vi "Disabled.vi"(7 "Robot Mode":T2, 10 "Match Info":T1={"Autonomous Elapsed Seconds"=0.0, "TeleOp Elapsed Seconds"=0.0, "Disabled Elapsed Seconds"=0.0, "Visited Autonomous"=FALSE, "Visited TeleOp"=FALSE, "Visited Disabled"=FALSE, "Autonomous Settings"={"Autonomous Style"=enum."Independent", "VI Refnum"=refnum}}, 11 "Call Context":T3) -> ()   [LabVIEW 2013]
doc: "This VI is called each time a disabled packet is received from the DS. It is often used to prepare for the next robot mode, to calibrate sensors, etc."
uses:
  <vilib>/Rock Robotics/WPI/DriverStation/WPI_DriverStationDerivedRobotMode.ctl
  <vilib>/Rock Robotics/WPI/DriverStation/WPI_DriverStationRobotMode2.ctl
  <vilib>/Rock Robotics/WPI/DriverStation/WPI_DriverStationMatch Info.ctl
  Systems/Catapult/Catapult.lvclass
  Systems/GrabberArms/GrabberArms.lvclass
  Systems/DriveMotors/DriveMotors.lvclass
  Robot Global Data.vi
panel:
  out "error out":errorcluster
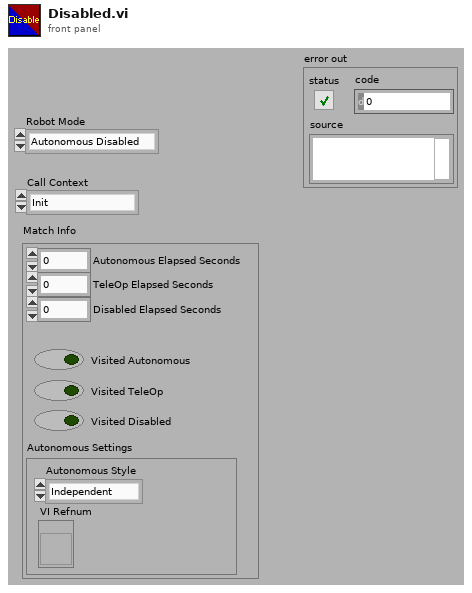
[diagram p1: front panel]
types:
  T1 = typedef "WPI_DriverStationMatch Info.ctl" = cluster{"Autonomous Elapsed Seconds":dbl, "TeleOp Elapsed Seconds":dbl, "Disabled Elapsed Seconds":dbl, "Visited Autonomous":bool, "Visited TeleOp":bool, "Visited Disabled":bool, "Autonomous Settings":cluster{"Autonomous Style":enum16{"Iterative", "Independent"}, "VI Refnum":refnum<vi>}}
  T2 = typedef "WPI_DriverStationRobotMode2.ctl" = enum16{"Autonomous Disabled", "Autonomous Enabled", "Teleop Disabled", "Teleop Enabled", "Timeout", "Finish", "Test Disabled", "Test Enabled"}
  T3 = typedef "WPI_DriverStationDerivedRobotMode.ctl" = enum16{"Init", "Execute", "Stop"}
  T4 = typedef "WPI_DriverStationAllianceInfo.ctl" = enum16{"Red", "Blue", "Invalid"}
  T5 = typedef "WPI_DigitalInputDevRef.ctl" = cluster{"DevStatus":errorcluster, "DIO Channel":T6, "Digital Module":T7}
  T6 = typedef "FPGA_DIOChannel.ctl" = enum8{"DIO 1", "DIO 2", "DIO 3", "DIO 4", "DIO 5", "DIO 6", "DIO 7", "DIO 8", "DIO 9", "DIO 10", "DIO 11", "DIO 12", "DIO 13", "DIO 14", "Invalid"}
  T7 = typedef "FPGA_TypedefDigitalModule.ctl" = enum16{"Digital Module 1", "Digital Module 2"}
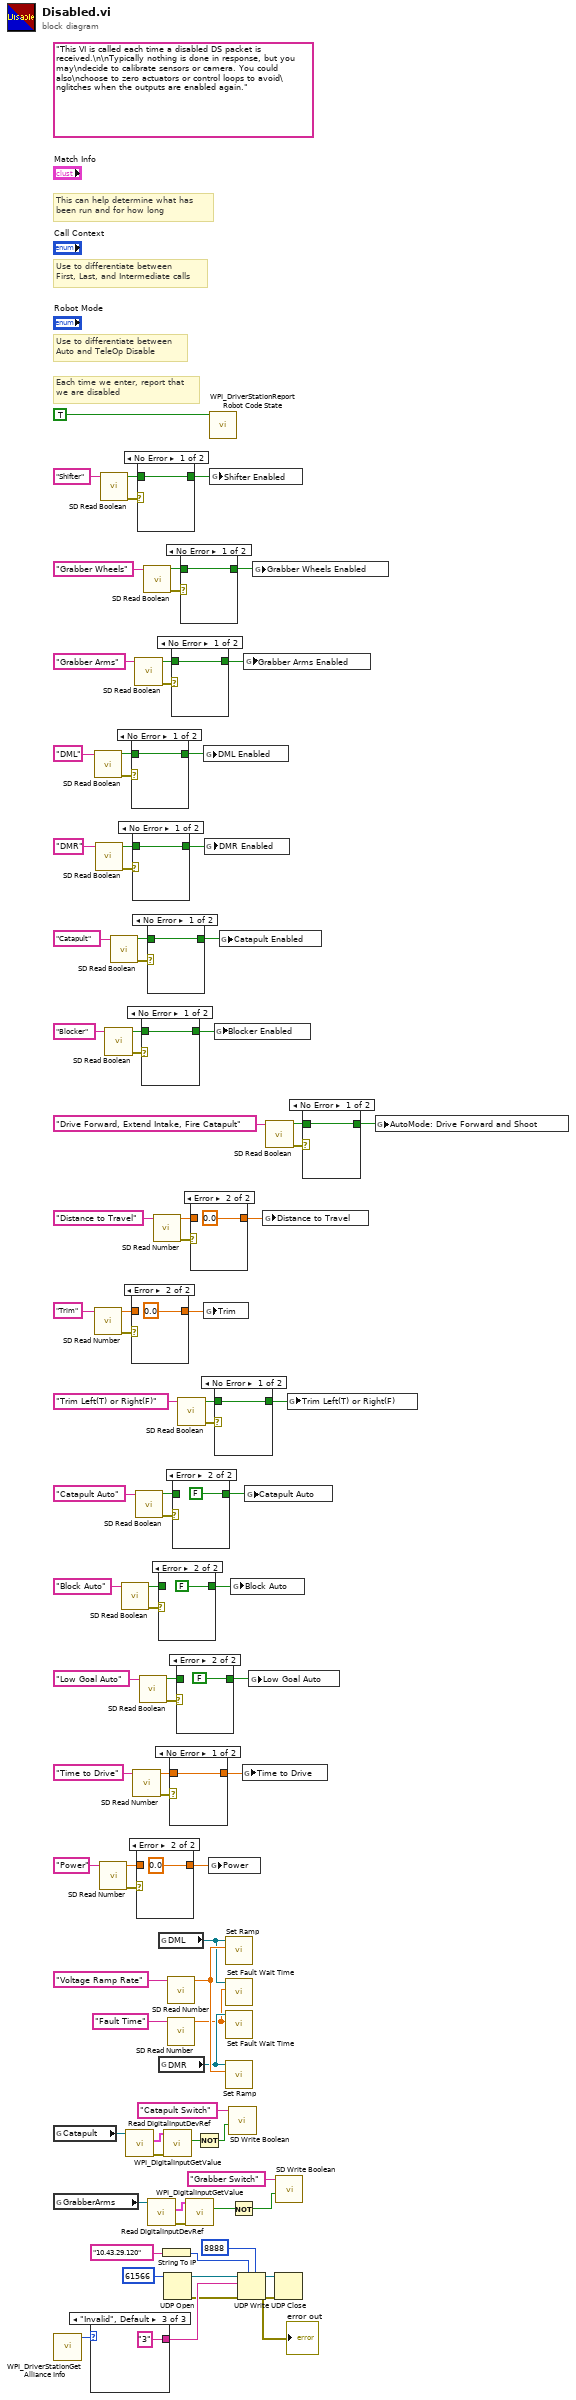
[diagram p0: block diagram]
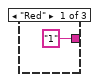
[diagram p2: hidden frame]
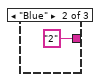
[diagram p3: hidden frame]
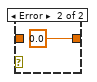
[diagram p8: hidden frame]
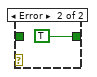
[diagram p9: hidden frame]
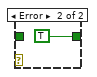
[diagram p12: hidden frame]
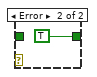
[diagram p13: hidden frame]
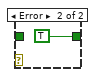
[diagram p14: hidden frame]
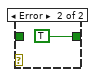
[diagram p15: hidden frame]
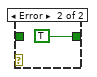
[diagram p16: hidden frame]
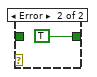
[diagram p17: hidden frame]
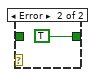
[diagram p18: hidden frame]
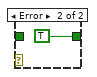
[diagram p19: hidden frame]
diagram:
  (unwired) "This VI is called each time a disabled DS packet is received.\n\nTypically nothing is done in response, but you may\ndecide to calibrate sensors or camera. You could also\nchoose to zero actuators or control loops to avoid\nglitches when the outputs are enabled again."
  # "Each time we enter, report that\nwe are disabled"
  # "Use to differentiate between\nFirst, Last, and Intermediate calls"
  # "This can help determine what has\nbeen run and for how long"
  # "Use to differentiate between\nAuto and TeleOp Disable"
  n1 = global read "Robot Global Data.vi" "Catapult"() -> (w39:refnum<class "Catapult.lvclass">)
  n2 = global read "Robot Global Data.vi" "GrabberArms"() -> (w5:refnum<class "GrabberArms.lvclass">)
  n3 = call <vilib>:"WPI_DriverStationGet Alliance Info.vi"() -> ("Alliance"=w11:T4)  [unwired: 10 in, 1 out]
  n4 = case shown="\"Invalid\", Default" w11 {
    tunnel: ["1" ("data in") "2" ("data in") "3" ("data in")] -> w10
    frame "Red" {
    }
    frame "Blue" {
    }
    frame "Invalid", Default {
    }
  }
  n5 = call <vilib>:"SD Read Boolean.vi"("Name"="DML") -> ("error out"=w83:errorcluster, "Boolean"=w74:bool)  [unwired: 8 in, 1 out]
  n6 = call <vilib>:"SD Read Number.vi"("Name"="Trim") -> ("error out"=w55:errorcluster, "Numeric"=w54:dbl)  [unwired: 8 in, 1 out]
  n7 = call <vilib>:"SD Read Boolean.vi"("Name"="DMR") -> ("error out"=w82:errorcluster, "Boolean"=w72:bool)  [unwired: 8 in, 1 out]
  n8 = call <vilib>:"SD Read Number.vi"("Name"="Power") -> ("error out"=w43:errorcluster, "Numeric"=w42:dbl)  [unwired: 8 in, 1 out]
  n9 = call <vilib>:"SD Read Boolean.vi"("Name"="Shifter") -> ("error out"=w86:errorcluster, "Boolean"=w80:bool)  [unwired: 8 in, 1 out]
  n10 = call <vilib>:"SD Read Boolean.vi"("Name"="Blocker") -> ("error out"=w66:errorcluster, "Boolean"=w67:bool)  [unwired: 8 in, 1 out]
  n11 = call <vilib>:"SD Read Boolean.vi"("Name"="Catapult") -> ("error out"=w81:errorcluster, "Boolean"=w70:bool)  [unwired: 8 in, 1 out]
  n12 = call <vilib>:"SD Read Boolean.vi"("Name"="Block Auto") -> ("error out"=w28:errorcluster, "Boolean"=w27:bool)  [unwired: 8 in, 1 out]
  n13 = call-dynamic "Read DigitalInputDevRef.vi"("Catapult in"=w39) -> ("error out"=w38:errorcluster, "DigitalInputDevRef"=w37:T5)  [unwired: 8 in, 1 out]
  n14 = case shown="No Error" w83 {
    tunnel: w74 -> [w97 _]
    tunnel: [w97 TRUE] -> w73
    frame No Error {
    }
    frame Error {
    }
  }
  n15 = case shown="Error" w55 {
    tunnel: [w99 0.0 ("Numeric")] -> w53
    tunnel: w54 -> [w99 _]
    frame No Error {
    }
    frame Error {
    }
  }
  n16 = case shown="No Error" w82 {
    tunnel: [w101 TRUE] -> w71
    tunnel: w72 -> [w101 _]
    frame No Error {
    }
    frame Error {
    }
  }
  n17 = call <vilib>:"SD Read Number.vi"("Name"="Time to Drive") -> ("error out"=w46:errorcluster, "Numeric"=w47:dbl)  [unwired: 8 in, 1 out]
  n18 = call <vilib>:"SD Read Boolean.vi"("Name"="Grabber Arms") -> ("error out"=w84:errorcluster, "Boolean"=w76:bool)  [unwired: 8 in, 1 out]
  n19 = call <vilib>:"SD Read Boolean.vi"("Name"="Catapult Auto") -> ("error out"=w23:errorcluster, "Boolean"=w24:bool)  [unwired: 8 in, 1 out]
  n20 = case shown="Error" w43 {
    tunnel: [w103 0.0 ("Numeric")] -> w41
    tunnel: w42 -> [w103 _]
    frame No Error {
    }
    frame Error {
    }
  }
  n21 = case shown="No Error" w86 {
    tunnel: w80 -> [w105 _]
    tunnel: [w105 TRUE] -> w79
    frame No Error {
    }
    frame Error {
    }
  }
  n22 = call <vilib>:"SD Read Boolean.vi"("Name"="Low Goal Auto") -> ("error out"=w20:errorcluster, "Boolean"=w19:bool)  [unwired: 8 in, 1 out]
  n23 = case shown="No Error" w66 {
    tunnel: [w107 TRUE] -> w68
    tunnel: w67 -> [w107 _]
    frame No Error {
    }
    frame Error {
    }
  }
  n24 = call <vilib>:"SD Read Boolean.vi"("Name"="Grabber Wheels") -> ("error out"=w85:errorcluster, "Boolean"=w78:bool)  [unwired: 8 in, 1 out]
  n25 = case shown="No Error" w81 {
    tunnel: [w109 TRUE] -> w69
    tunnel: w70 -> [w109 _]
    frame No Error {
    }
    frame Error {
    }
  }
  n26 = call-dynamic "Read DigitalInputDevRef.vi"("GrabberArms in"=w5) -> ("error out"=w32:errorcluster, "DigitalInputDevRef"=w33:T5)  [unwired: 8 in, 1 out]
  n27 = call <vilib>:"SD Read Number.vi"("Name"="Distance to Travel") -> ("error out"=w59:errorcluster, "Numeric"=w58:dbl)  [unwired: 8 in, 1 out]
  n28 = case shown="Error" w28 {
    tunnel: [w111 FALSE] -> w26
    tunnel: w27 -> [w111 _]
    frame No Error {
    }
    frame Error {
    }
  }
  n29 = global read "Robot Global Data.vi" "DML"() -> (w13:refnum<class "DriveMotors.lvclass">)
  n30 = global read "Robot Global Data.vi" "DMR"() -> (w14:refnum<class "DriveMotors.lvclass">)
  n31 = String To IP(1:"10.43.29.120" ("name")) -> (0:w7:u32)
  n32 = call <vilib>:"WPI_DigitalInputGetValue.vi"("error in (no error)"=w38, "DigitalInputDevRef"=w37) -> ("Value"=w36:bool)  [unwired: 7 in, 2 out]
  n33 = UDP Open(11:u16 61566 ("port")) -> (port=w6:refnum<k16>, 0:w1:errorcluster)  [unwired: 4 in, 1 out]
  n34 = call <vilib>:"SD Read Number.vi"("Name"="Voltage Ramp Rate") -> ("Numeric"=w16:dbl)  [unwired: 8 in, 2 out]
  n35 = call <vilib>:"SD Read Number.vi"("Name"="Fault Time") -> ("Numeric"=w12:dbl)  [unwired: 8 in, 2 out]
  n36 = case shown="No Error" w46 {
    tunnel: [w113 0.0 ("Numeric")] -> w48
    tunnel: w47 -> [w113 _]
    frame No Error {
    }
    frame Error {
    }
  }
  n37 = case shown="No Error" w84 {
    tunnel: w76 -> [w115 _]
    tunnel: [w115 TRUE] -> w75
    frame No Error {
    }
    frame Error {
    }
  }
  n38 = case shown="Error" w23 {
    tunnel: [w117 FALSE] -> w25
    tunnel: w24 -> [w117 _]
    frame No Error {
    }
    frame Error {
    }
  }
  n39 = case shown="Error" w20 {
    tunnel: [w119 FALSE] -> w18
    tunnel: w19 -> [w119 _]
    frame No Error {
    }
    frame Error {
    }
  }
  n40 = call <vilib>:"SD Read Boolean.vi"("Name"="Trim Left(T) or Right(F)") -> ("error out"=w50:errorcluster, "Boolean"=w51:bool)  [unwired: 8 in, 1 out]
  n41 = case shown="No Error" w85 {
    tunnel: w78 -> [w121 _]
    tunnel: [w121 TRUE] -> w77
    frame No Error {
    }
    frame Error {
    }
  }
  n42 = call <vilib>:"WPI_DigitalInputGetValue.vi"("error in (no error)"=w32, "DigitalInputDevRef"=w33) -> ("Value"=w35:bool)  [unwired: 7 in, 2 out]
  n43 = case shown="Error" w59 {
    tunnel: [w123 0.0 ("Numeric")] -> w57
    tunnel: w58 -> [w123 _]
    frame No Error {
    }
    frame Error {
    }
  }
  n44 = Not(x=w36) -> (.not. x?=w31:bool)
  n45 = global write "Robot Global Data.vi" "DML Enabled"(w73) -> ()
  n46 = global write "Robot Global Data.vi" "Trim"(w53) -> ()
  n47 = global write "Robot Global Data.vi" "DMR Enabled"(w71) -> ()
  n48 = global write "Robot Global Data.vi" "Power"(w41) -> ()
  n49 = call <vilib>:"WPI_DriverStationReport Robot Code State.vi"("Disabled"=TRUE ("Autonomous")) -> ()  [unwired: 10 in, 1 out]
  n50 = global write "Robot Global Data.vi" "Shifter Enabled"(w79) -> ()
  n51 = global write "Robot Global Data.vi" "Blocker Enabled"(w68) -> ()
  n52 = case shown="No Error" w50 {
    tunnel: [w125 TRUE] -> w52
    tunnel: w51 -> [w125 _]
    frame No Error {
    }
    frame Error {
    }
  }
  n53 = global write "Robot Global Data.vi" "Catapult Enabled"(w69) -> ()
  n54 = call-dynamic "Set Ramp.vi"("VoltageRampRate (V/s)"=w16, "DriveMotors in"=w13) -> ()  [unwired: 8 in, 2 out]
  n55 = call-dynamic "Set Fault Wait Time.vi"("Fault Time(s)"=w12, "DriveMotors in"=w13) -> ()  [unwired: 8 in, 2 out]
  n56 = call-dynamic "Set Fault Wait Time.vi"("Fault Time(s)"=w12, "DriveMotors in"=w14) -> ()  [unwired: 8 in, 2 out]
  n57 = call-dynamic "Set Ramp.vi"("VoltageRampRate (V/s)"=w16, "DriveMotors in"=w14) -> ()  [unwired: 8 in, 2 out]
  n58 = call <vilib>:"SD Write Boolean.vi"("Boolean"=w31, "Name"="Catapult Switch") -> ()  [unwired: 8 in, 2 out]
  n59 = Not(x=w35) -> (.not. x?=w30:bool)
  n60 = global write "Robot Global Data.vi" "Block Auto"(w26) -> ()
  n61 = UDP Write(address=w7, port or service name=u16 8888 ("port"), connection ID=w6, data in=w10, 8:w1) -> (error out=w8:errorcluster, 3:w9:refnum<k16>)  [unwired: 1 in]
  "error out" <- w8
  n62 = global write "Robot Global Data.vi" "Time to Drive"(w48) -> ()
  n63 = global write "Robot Global Data.vi" "Grabber Arms Enabled"(w75) -> ()
  n64 = global write "Robot Global Data.vi" "Catapult Auto"(w25) -> ()
  n65 = global write "Robot Global Data.vi" "Low Goal Auto"(w18) -> ()
  n66 = global write "Robot Global Data.vi" "Grabber Wheels Enabled"(w77) -> ()
  n67 = global write "Robot Global Data.vi" "Distance to Travel"(w57) -> ()
  n68 = call <vilib>:"SD Read Boolean.vi"("Name"="Drive Forward, Extend Intake, Fire Catapult") -> ("error out"=w63:errorcluster, "Boolean"=w62:bool)  [unwired: 8 in, 1 out]
  n69 = UDP Close(connection ID=w9, 8:w8) -> ()  [unwired: 2 out]
  n70 = call <vilib>:"SD Write Boolean.vi"("Boolean"=w30, "Name"="Grabber Switch") -> ()  [unwired: 8 in, 2 out]
  n71 = global write "Robot Global Data.vi" "Trim Left(T) or Right(F)"(w52) -> ()
  n72 = case shown="No Error" w63 {
    tunnel: [w127 TRUE] -> w61
    tunnel: w62 -> [w127 _]
    frame No Error {
    }
    frame Error {
    }
  }
  n73 = global write "Robot Global Data.vi" "AutoMode: Drive Forward and Shoot"(w61) -> ()
